vi "OAT Output Trigger Event (XY).vi"(0 "signal in":cluster{"X":dbl[], "Y":dbl[]} {"X" format="%.2f"; "Y" format="%.2f"}, 1 "trigger on":T1(ring), 2 "reset? (F)":bool, 5 "upper setpoint":dbl=inf, 7 "lower setpoint":dbl=-inf, 9 "hysteresis":dbl format="%.2p", 11 "error in (no error)":errorcluster) -> (4 "trigger detected?":bool, 15 "error out":errorcluster)   [LabVIEW 2017, in "SoundVib_OAUtility.lvlib"]
doc: "Detects the first level-crossing condition. The <B>upper setpoint</B> and <B>lower setpoint</B> of the threshold and the <B>hysteresis</B> specify the trigger conditions. Wire data to the <B>signal in</B> input to determine the polymorphic instance to use or manually select the instance."
uses:
  <vilib>/addons/Sound and Vibration/Order Analysis/Utility/SoundVib_OAUtility.lvlib
  <vilib>/measure/mamon.llb/Trigger Detection for 1 Channel.vi
  <vilib>/measure/NI_MAPro.lvlib
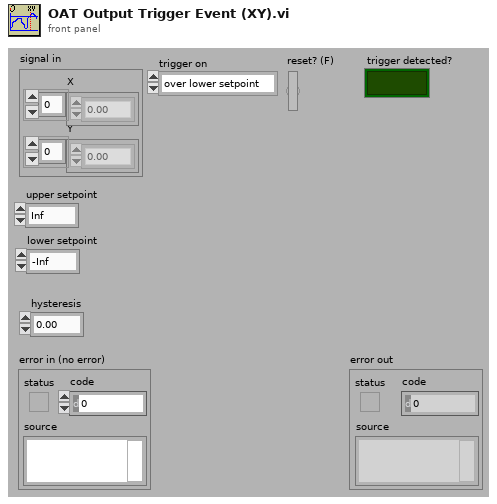
[diagram p1: front panel]
types:
  T1 = enum16{"over lower setpoint", "under upper setpoint", "both"}
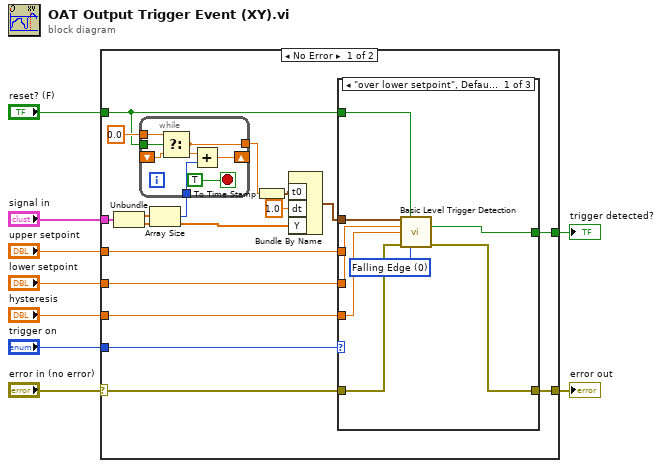
[diagram p0: block diagram]
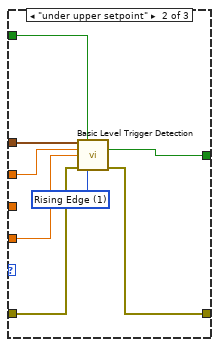
[diagram p2: hidden frame]
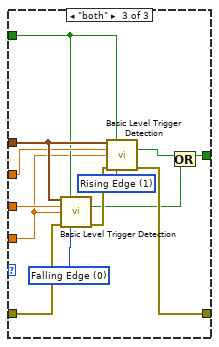
[diagram p3: hidden frame]
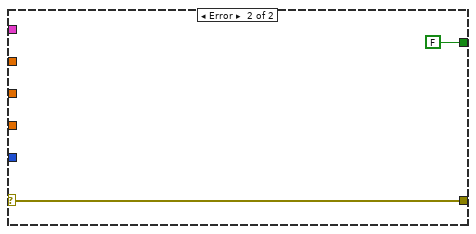
[diagram p4: hidden frame]
diagram:
  n1 = case shown="No Error" "error in (no error)" {
    selector: "error in (no error)" -> [w21 w64]
    tunnel: [w20 w64] -> w8
    tunnel: "signal in" -> [w26 _]
    tunnel: "upper setpoint" -> [w25 _]
    tunnel: "lower setpoint" -> [w24 _]
    tunnel: "hysteresis" -> [w23 _]
    tunnel: "trigger on" -> [w22 _]
    tunnel: [w19 FALSE ("trigger detected?")] -> w2
    tunnel: "reset? (F)" -> [w17 _]
    frame No Error {
      n2 = Unbundle(w26) -> ("X"=w16:dbl[], "Y"=w14:dbl[])
      n3 = Array Size(array=w16) -> (size(s)=w15:i32)
      n4 = while {
        shift-right: [w28] -> _
        shift-left: _ -> [w30]
        tunnel: 0.0 ("t") -> [w32]
        tunnel: w17 -> [w31]
        tunnel: w15 -> [w29]
        tunnel: [w27] -> w12
        stop <- TRUE stop-if-true
        n5 = Select(t=w32, s=w31, f=w30) -> (s? t:f=w27:dbl)
        n6 = Add(x=w27, y=w29) -> (x+y=w28:dbl)
      }
      n7 = To Time Stamp(1:w12) -> (0:w11:timestamp)
      n8 = Bundle By Name("t0"=w11, "dt"=1.0, "Y"=w14) -> (w10:waveform(dbl))  [unwired: 1 in]
      n9 = case shown="\"over lower setpoint\", Default" w22 {
        tunnel: w10 -> [w41 w49 w62]
        tunnel: w17 -> [w40 w48 w51]
        tunnel: w24 -> [w38 _ w60]
        tunnel: w21 -> [w37 w46 w57]
        tunnel: [w36 w43 w55] -> w20
        tunnel: [w35 w44 w52] -> w19
        tunnel: w25 -> [_ w47 w61]
        tunnel: w23 -> [w34 w42 w50]
        frame "over lower setpoint", Default {
          w39 = u16 0 items=["Falling Edge", "Rising Edge"] ("slope")
          n10 = call-poly <vilib>:"Basic Level Trigger Detection.vi"("signal in"=w41, "reset"=w40, "level"=w38, "hysteresis"=w34, "error in (no error)"=w37, "trigger slope"=w39) -> ("trigger detected?"=w35:bool, "error out"=w36:errorcluster)  [unwired: 7 in, 1 out]
        }
        frame "under upper setpoint" {
          w45 = u16 1 items=["Falling Edge", "Rising Edge"] ("slope")
          n11 = call-poly <vilib>:"Basic Level Trigger Detection.vi"("signal in"=w49, "reset"=w48, "level"=w47, "hysteresis"=w42, "error in (no error)"=w46, "trigger slope"=w45) -> ("trigger detected?"=w44:bool, "error out"=w43:errorcluster)  [unwired: 7 in, 1 out]
        }
        frame "both" {
          w58 = u16 0 items=["Falling Edge", "Rising Edge"] ("slope")
          w59 = u16 1 items=["Falling Edge", "Rising Edge"] ("slope")
          n12 = call-poly <vilib>:"Basic Level Trigger Detection.vi"("signal in"=w62, "reset"=w51, "level"=w60, "hysteresis"=w50, "error in (no error)"=w57, "trigger slope"=w58) -> ("trigger detected?"=w53:bool, "error out"=w56:errorcluster)  [unwired: 7 in, 1 out]
          n13 = call-poly <vilib>:"Basic Level Trigger Detection.vi"("signal in"=w62, "reset"=w51, "level"=w61, "hysteresis"=w50, "error in (no error)"=w56, "trigger slope"=w59) -> ("trigger detected?"=w54:bool, "error out"=w55:errorcluster)  [unwired: 7 in, 1 out]
          n14 = Or(x=w54, y=w53) -> (x .or. y?=w52:bool)
        }
      }
    }
    frame Error {
    }
  }
  "error out" <- w8
  "trigger detected?" <- w2
